vi "TopLevel.vi"(10 "Ad-Hoc Installers":T4 {"MachineName" items=["Machine-01", "Machine-02", "Machine-03", "Machine-04", "Machine-05", "Machine-06", "Machine-07", "Machine-08", "Machine-09", "Machine-10", "Machine-11", "Machine-12", "Machine-13", "Machine-14", "Machine-15", "Machine-16"]}, 11 "Latest installers":T3 {"Machine Name" items=["Machine-01", "Machine-02", "Machine-03", "Machine-04", "Machine-05", "Machine-06", "Machine-07", "Machine-08", "Machine-09", "Machine-10", "Machine-11", "Machine-12", "Machine-13", "Machine-14", "Machine-15", "Machine-16"]; "Branch-CSDS" items=["R3-Bitness[NI]", "R3-Releases-CSDS[NI]", "R3-RFC-Main[NI]", "R3-SD-Main[NI]", "R3-Trunk[NI]", "R3-VI-Main[NI]"]; "Branch-LVMD" items=["R2-Releases-LVMD[NI]", "R2-Releases-MCC[NI]"]}) -> ()   [LabVIEW 2013]
uses:
  ControlAd-Hoc.ctl
  MachineNames.ctl
  ControlLatestInstall.ctl
  ControlBranchName.ctl
  <vilib>/smtpClient/Set Message Text Html.vi
  <vilib>/Utility/config.llb/NI_LVConfig.lvlib
  <vilib>/smtpClient/LabVIEWSMTPClient.lvlib
panel:
  in  "Minutes to wait":u32
  in  "EMAIL LIST":string[](array[string])
  out "Branch-CSDS 1":T1 items=["R3-Bitness[NI]", "R3-Releases-CSDS[NI]", "R3-RFC-Main[NI]", "R3-SD-Main[NI]", "R3-Trunk[NI]", "R3-VI-Main[NI]"]
  out "Branch-LVMD 1":T1 items=["R2-Releases-LVMD[NI]", "R2-Releases-MCC[NI]"]
  out "Machine Name 1":T2=3 items=["Machine-01", "Machine-02", "Machine-03", "Machine-04", "Machine-05", "Machine-06", "Machine-07", "Machine-08", "Machine-09", "Machine-10", "Machine-11", "Machine-12", "Machine-13", "Machine-14", "Machine-15", "Machine-16"]
  in  "path":path=path "\\\\nibataserver\\Reports/NG/Manual Testing"
  in  "FLUSH Old Scripts":bool
  in  "Path to search Branches CSDS":path=path "\\\\in-ban-argo.natinst.com\\NISoftwarePrerelease/LabVIEW Communications System Design Suite/R3-Altair/Daily"
  in  "Path to search Branches LVMD":path=path "\\\\in-ban-argo.natinst.com\\NISoftwarePrerelease/LabVIEW for myDAQ/1.0/Daily"
  in  "OK Button":bool
  in  "Ring":u16(ring) items=["Install Latest", "Install Ad-Hoc"]
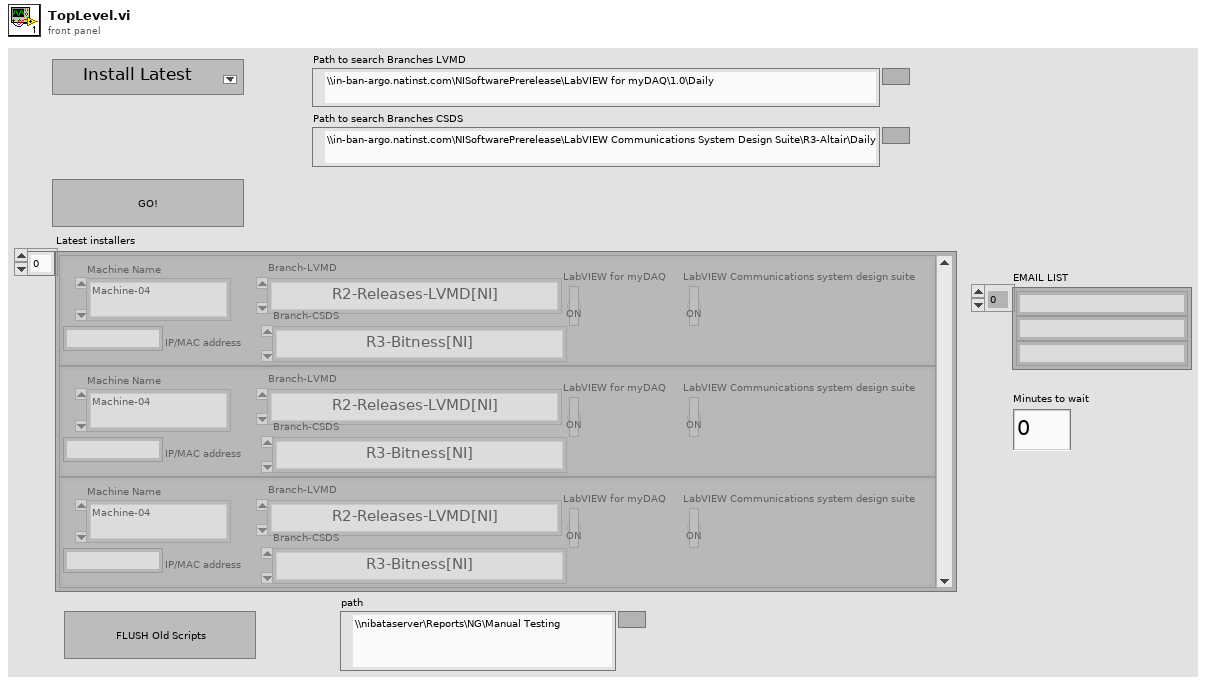
[diagram p1: front panel]
types:
  T1 = typedef "ControlBranchName.ctl" = u16
  T2 = typedef "MachineNames.ctl" = u16
  T3 = typedef "ControlLatestInstall.ctl" = cluster{"Branch-LVMD":T1, "LabVIEW for myDAQ":bool, "LabVIEW Communications system design suite":bool, "IP/MAC address":string, "Branch-CSDS":T1, "Machine Name":T2}[]
  T4 = typedef "ControlAd-Hoc.ctl" = cluster{"Installer Array":path[], "MachineName":T2, "IP/MAC Add":string}[]
  T5 = typedef "NI_LVConfig.lvlib/Config Data RefNum.ctl" = refnum<k1>
  T6 = typedef "LabVIEWSMTPClient.lvlib/SmtpClientHandle.ctl" = refnum<k1>
  T7 = enum16{"Left Button", "Center Button", "Right Button", "Window Close"}
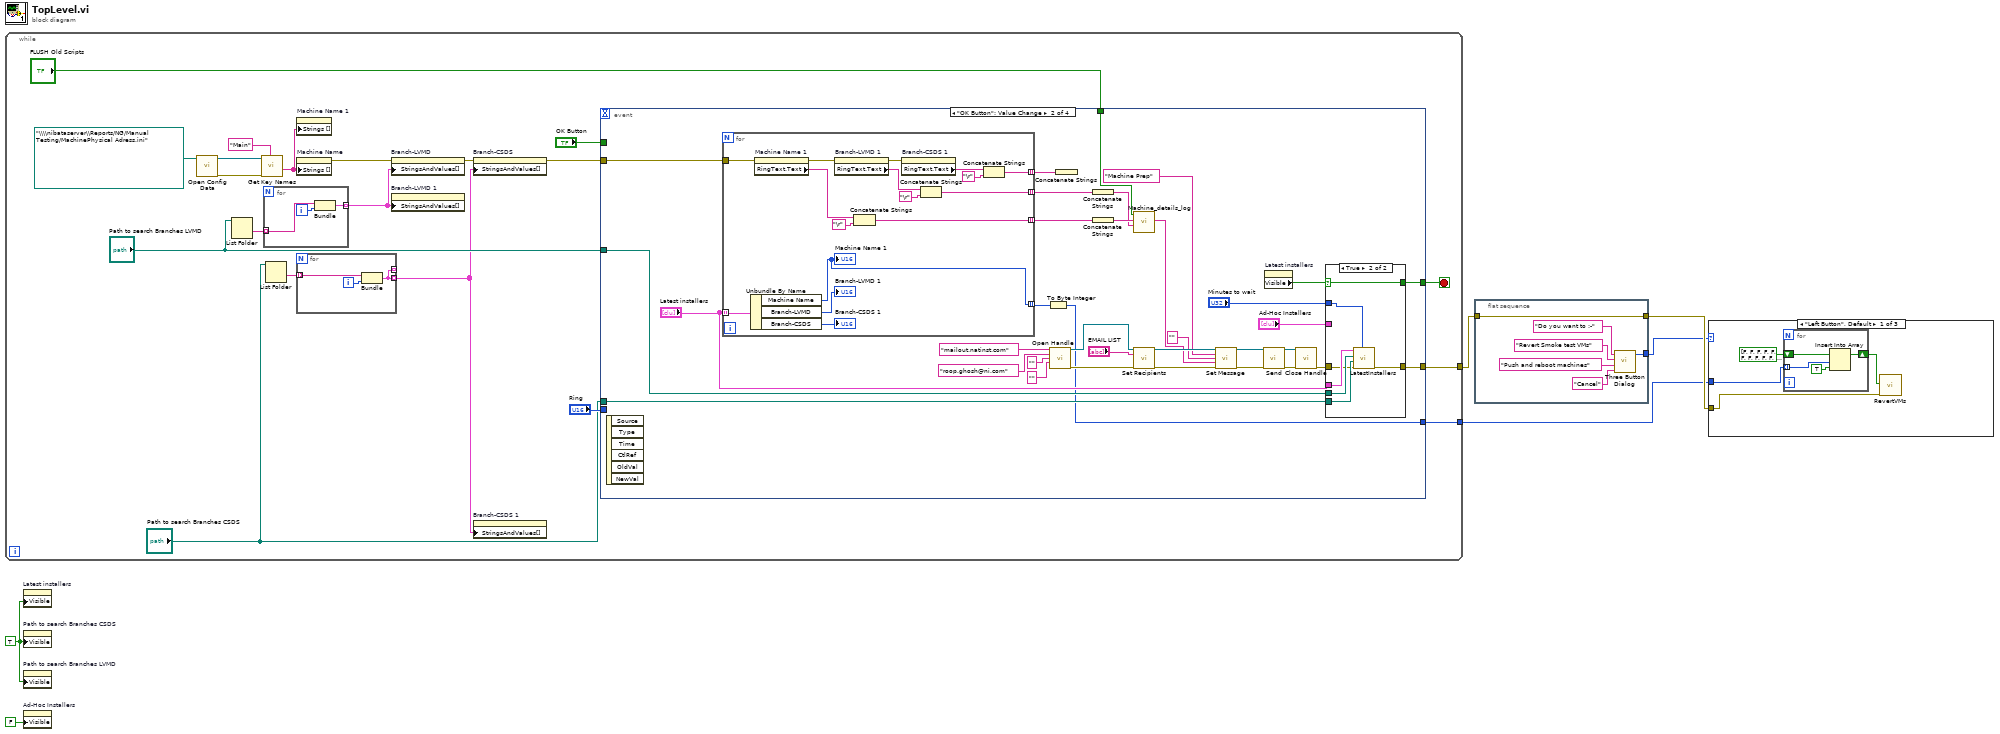
[diagram p0: block diagram]
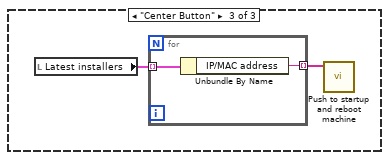
[diagram p3: hidden frame]
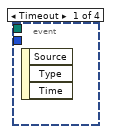
[diagram p4: hidden frame]
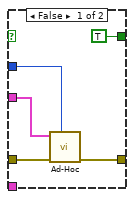
[diagram p5: hidden frame]
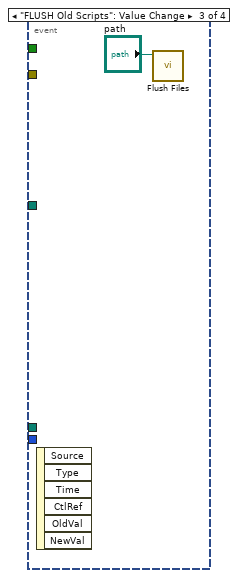
[diagram p6: hidden frame]
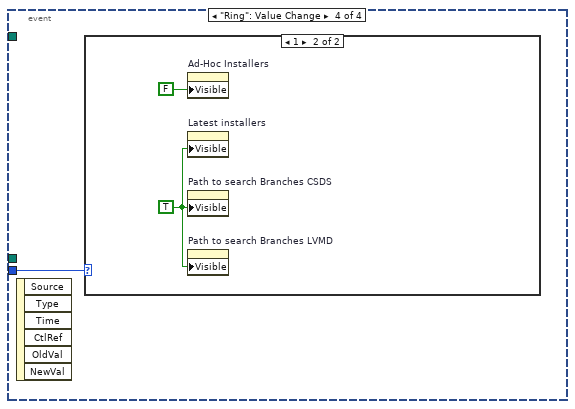
[diagram p7: hidden frame]
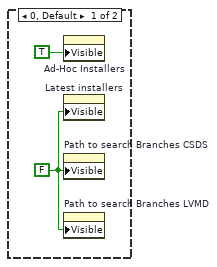
[diagram p8: hidden frame]
diagram:
  w5 = TRUE ("Visible")
  n1 = while {
    tunnel: [w22] -> w4
    tunnel: [w7] -> w1
    stop <- w23 stop-if-true
    n2 = call <vilib>:"Open Config Data.vi"("configuration file path"=path "\\\\nibataserver\\Reports/NG/Manual Testing/MachinePhysical Adress.ini") -> ("error out"=w18:errorcluster, "refnum"=w20:T5)  [unwired: 8 in, 1 out]
    n3 = List Folder(path="Path to search Branches LVMD") -> (folder names=w24:string[])  [unwired: 3 in, 3 out]
    n4 = call <vilib>:"Get Key Names.vi"("section"="Main", "error in (no error)"=w18, "refnum"=w20) -> ("key names"=w11:string[])  [unwired: 5 in, 3 out]
    n5 = for {
      tunnel: w24 -> [w32] mode=indexing
      tunnel: [w30] -> w10 mode=indexing
      i -> [w31]
      n6 = Bundle(w32, w31) -> (w30:cluster{string, i32})  [unwired: 1 in]
    }
    n7 = List Folder(path="Path to search Branches CSDS") -> (folder names=w16:string[])  [unwired: 3 in, 3 out]
    n8 = property on="Machine Name 1" class="Ring (strict)"("Strings []"=w11) -> ()  [unwired: 2 in, 2 out]
    n9 = property on="Machine Name" class="Ring (strict)"("Strings []"=w11) -> (error out=w14:errorcluster)  [unwired: 2 in, 1 out]
    n10 = for {
      tunnel: w16 -> [w29] mode=indexing
      tunnel: [w27] -> _ mode=indexing
      tunnel: [w27] -> w9 mode=indexing
      i -> [w28]
      n11 = Bundle(w29, w28) -> (w27:cluster{string, i32})  [unwired: 1 in]
    }
    n12 = property on="Branch-LVMD" class="Ring (strict)"(error in=w14, "StringsAndValues[]"=w10) -> (error out=w13:errorcluster)  [unwired: 1 in, 1 out]
    n13 = property on="Branch-LVMD 1" class="Ring (strict)"("StringsAndValues[]"=w10) -> ()  [unwired: 2 in, 2 out]
    n14 = property on="Branch-CSDS" class="Ring (strict)"(error in=w13, "StringsAndValues[]"=w9) -> (error out=w12:errorcluster)  [unwired: 1 in, 1 out]
    n15 = property on="Branch-CSDS 1" class="Ring (strict)"("StringsAndValues[]"=w9) -> ()  [unwired: 2 in, 2 out]
    n16 = event shown="[1] \"OK Button\": Value Change" {
      selector: _ -> [_ _ _ _]
      dyn-events: _ -> [_ _ _ _]
      timeout: _ -> [_ _ _ _]
      tunnel: "OK Button" -> [_ _ _ _]
      tunnel: "Ring" -> [_ _ _ w96]
      tunnel: [_ w65 _ _] -> w23
      tunnel: [_ w64 _ _] -> w22
      tunnel: "Path to search Branches LVMD" -> [_ w63 _ _]
      tunnel: "Path to search Branches CSDS" -> [_ w62 _ _]
      tunnel: w12 -> [_ w59 _ _]
      tunnel: "FLUSH Old Scripts" -> [_ w36 _ _]
      tunnel: [_ w34 _ _] -> w7
      event Timeout {
        n17 = event-data() -> ()  [unwired: 1 in, 3 out]
      }
      event "OK Button": Value Change {
        n18 = event-data() -> ()  [unwired: 1 in, 6 out]
        n19 = for {
          tunnel: "Latest installers" -> [w82] mode=indexing
          tunnel: w59 -> [w79]
          tunnel: [w74] -> w58 mode=indexing
          tunnel: [w72] -> w57 mode=indexing
          tunnel: [w68] -> w56 mode=indexing
          tunnel: [w67] -> w35 mode=indexing
          n20 = Unbundle By Name(w82) -> ("Machine Name"=w67:T2, "Branch-LVMD"=→"Branch-LVMD 1":T1, "Branch-CSDS"=→"Branch-CSDS 1":T1)
          "Machine Name 1" <- w67
          n21 = property on="Machine Name 1" class="Ring (strict)"(error in=w79) -> (error out=w78:errorcluster, "RingText.Text"=w75:string)  [unwired: 1 in, 1 out]
          n22 = property on="Branch-LVMD 1" class="Ring (strict)"(error in=w78) -> (error out=w77:errorcluster, "RingText.Text"=w73:string)  [unwired: 1 in, 1 out]
          n23 = Concatenate Strings(w75, "\r") -> (w74:string)
          n24 = property on="Branch-CSDS 1" class="Ring (strict)"(error in=w77) -> ("RingText.Text"=w69:string)  [unwired: 1 in, 2 out]
          n25 = Concatenate Strings(w73, "\r") -> (w72:string)
          n26 = Concatenate Strings(w69, "\r") -> (w68:string)
        }
        n27 = To Byte Integer(number=w35) -> (8bit integer=w34:i8[])
        n28 = call <vilib>:"Open Handle.vi"("server address"="mailout.natinst.com", "from"="roop.ghosh@ni.com", "username"="", "password"="") -> ("handle out"=w51:T6, "error out"=w41:errorcluster)  [unwired: 10 in]
        n29 = Concatenate Strings(w56) -> ()  [unwired: 1 out]
        n30 = Concatenate Strings(w57) -> (w54:string)
        n31 = Concatenate Strings(w58) -> (w55:string)
        n32 = call "Machine_details_log.vi"("Delete Old data?"=w36, "Machine name"=w55, "Branch Name"=w54) -> ("HTML TEXT"=w42:string)  [unwired: 1 in, 4 out]
        n33 = call <vilib>:"Set Recipients.vi"("handle in"=w51, "to"="EMAIL LIST", "error in (no error)"=w41) -> ("handle out"=w52:T6, "error out"=w40:errorcluster)  [unwired: 11 in]
        n34 = call-poly <vilib>:"Set Message.vi"("handle in"=w52, "subject"="Machine Prep" ("subject ([No Subject])"), "plain text message"="", "html message"=w42, "error in (no error)"=w40) -> ("handle out"=w50:T6, "error out"=w39:errorcluster)  [unwired: 9 in]
        n35 = call <vilib>:"Send.vi"("handle in"=w50, "error in (no error)"=w39) -> ("handle out"=w49:T6, "error out"=w38:errorcluster)  [unwired: 11 in, 1 out]
        n36 = property on="Latest installers" class="Arr (strict)"() -> ("Visible"=w66:bool)  [unwired: 2 in, 2 out]
        n37 = call <vilib>:"Close Handle.vi"("handle in"=w49, "error in (no error)"=w38) -> ("error out"=w37:errorcluster)  [unwired: 12 in, 1 out]
        n38 = case shown="True" w66 {
          selector: w66 -> [_ w94]
          tunnel: [TRUE w94] -> w65
          tunnel: [w86 w93] -> w64
          tunnel: w63 -> [_ w92]
          tunnel: w62 -> [_ w91]
          tunnel: "Ad-Hoc Installers" -> [w85 _]
          tunnel: "Latest installers" -> [_ w90]
          tunnel: w37 -> [w84 w89]
          tunnel: "Minutes to wait" -> [w83 w88]
          frame False {
            n39 = call "Ad-Hoc.vi"("Minutes to wait"=w83, "error in"=w84, "Ad-Hoc Installers"=w85) -> ("error Out"=w86:errorcluster)  [unwired: 7 in, 1 out]
          }
          frame True {
            n40 = call "LatestInstallers.vi"("Minutes to wait"=w88, "error in"=w89, "path to search latest folder CSDS"=w91, "path to search latest folder LVMD"=w92, "Latest installers"=w90) -> ("error out"=w93:errorcluster)  [unwired: 6 in]
          }
        }
      }
      event "FLUSH Old Scripts": Value Change {
        n41 = event-data() -> ()  [unwired: 1 in, 6 out]
        n42 = call "Flush Files.vi"("path"="path") -> ()  [unwired: 11 in]
      }
      event "Ring": Value Change {
        n43 = event-data() -> ()  [unwired: 1 in, 6 out]
        n44 = case shown="1" w96 {
          frame 0, Default {
            w97 = FALSE ("Visible")
            n45 = property on="Ad-Hoc Installers" class="Arr (strict)"("Visible"=TRUE) -> ()  [unwired: 2 in, 2 out]
            n46 = property on="Latest installers" class="Arr (strict)"("Visible"=w97) -> ()  [unwired: 2 in, 2 out]
            n47 = property on="Path to search Branches CSDS" class="Path"("Visible"=w97) -> ()  [unwired: 2 in, 2 out]
            n48 = property on="Path to search Branches LVMD" class="Path"("Visible"=w97) -> ()  [unwired: 2 in, 2 out]
          }
          frame 1 {
            w99 = TRUE ("Visible")
            n49 = property on="Ad-Hoc Installers" class="Arr (strict)"("Visible"=FALSE) -> ()  [unwired: 2 in, 2 out]
            n50 = property on="Latest installers" class="Arr (strict)"("Visible"=w99) -> ()  [unwired: 2 in, 2 out]
            n51 = property on="Path to search Branches CSDS" class="Path"("Visible"=w99) -> ()  [unwired: 2 in, 2 out]
            n52 = property on="Path to search Branches LVMD" class="Path"("Visible"=w99) -> ()  [unwired: 2 in, 2 out]
          }
        }
      }
    }
  }
  n53 = property on="Latest installers" class="Arr (strict)"("Visible"=w5) -> ()  [unwired: 2 in, 2 out]
  n54 = property on="Path to search Branches CSDS" class="Path"("Visible"=w5) -> ()  [unwired: 2 in, 2 out]
  n55 = property on="Path to search Branches LVMD" class="Path"("Visible"=w5) -> ()  [unwired: 2 in, 2 out]
  n56 = property on="Ad-Hoc Installers" class="Arr (strict)"("Visible"=FALSE) -> ()  [unwired: 2 in, 2 out]
  n57 = flat-sequence {
    tunnel: w4 -> [w106]
    tunnel: [w106] -> w3
    tunnel: [w101] -> w2
    frame #0 {
      n58 = call <vilib>:"Three Button Dialog.vi"("Right Button Text (\"Cancel\")"="Cancel" ("Right Button Text (\"Cancel\")"), "Center Button Text (\"No\")"="Push and reboot machines" ("F button name (\"Cancel\")"), "Left Button Text (\"Yes\")"="Revert Smoke test VMs" ("T button name (\"OK\")"), "message"="Do you want to :-") -> ("Which Button?"=w101:T7)  [unwired: 7 in]
    }
  }
  n59 = case shown="\"Left Button\", Default" w2 {
    tunnel: w3 -> [w108 _ _]
    tunnel: w1 -> [w107 _ _]
    frame "Left Button", Default {
      n60 = for {
        shift-right: [w113] -> w109
        shift-left: bool[] [FALSE, FALSE, FALSE, FALSE, FALSE, FALSE, FALSE, FALSE, FALSE, FALSE, FALSE, FALSE, FALSE, FALSE, FALSE, FALSE, FALSE, FALSE, FALSE, FALSE, TRUE, FALSE, FALSE, FALSE, FALSE, FALSE, FALSE, FALSE, FALSE, FALSE, FALSE, FALSE, FALSE, FALSE, FALSE, FALSE, FALSE, FALSE, FALSE, FALSE, FALSE, FALSE, FALSE, FALSE, FALSE, FALSE, FALSE, FALSE, FALSE, FALSE, FALSE, FALSE, FALSE, FALSE, FALSE, FALSE, FALSE, FALSE, FALSE, FALSE, FALSE, FALSE, FALSE, FALSE, FALSE, FALSE, FALSE, FALSE, FALSE, FALSE, FALSE, FALSE, FALSE, FALSE, FALSE, FALSE, FALSE, FALSE, FALSE, FALSE, FALSE, FALSE, FALSE, FALSE, FALSE, FALSE, FALSE, FALSE, FALSE, FALSE, FALSE, FALSE, FALSE, FALSE, FALSE, FALSE, FALSE, FALSE, FALSE, FALSE, FALSE, FALSE, FALSE, FALSE, FALSE, FALSE, FALSE, FALSE, FALSE, FALSE, FALSE, FALSE, FALSE, FALSE, FALSE, FALSE, FALSE, FALSE, FALSE, FALSE, FALSE, FALSE, FALSE, FALSE, FALSE, FALSE, FALSE, FALSE, FALSE, FALSE, FALSE, FALSE, FALSE, FALSE, FALSE, FALSE, FALSE, FALSE, FALSE, FALSE, FALSE, FALSE, FALSE, FALSE, FALSE, FALSE, FALSE, FALSE, FALSE, FALSE, TRUE] -> [w114]
        tunnel: w107 -> [w111] mode=indexing
        n61 = Insert Into Array(array=w114, index=w111, new element=TRUE ("new element/subarray")) -> (w113:bool[])
      }
      n62 = call "RevertVMs.vi"("error in (no error)"=w108, "Array"=w109) -> ()  [unwired: 9 in, 1 out]
    }
    frame "Right Button" {
    }
    frame "Center Button" {
      n63 = local read "Latest installers"() -> (w116:T3)
      n64 = for {
        tunnel: w116 -> [w118] mode=indexing
        tunnel: [w117] -> w115 mode=indexing
        n65 = Unbundle By Name(w118) -> ("IP/MAC address"=w117:string)
      }
      n66 = call "Push to startup and reboot machine.vi"("Array"=w115) -> ()  [unwired: 11 in]
    }
  }
